vi "Multiple Connections - Server - TCP - 複製 (2).vi"() -> ()   [LabVIEW 2011]
doc: "Demonstrates how to establish multiple connections and place them in a queue to be serviced. As connections are made, it sends the current date and time via TCP to all Client VIs that connect to it.\n\nThis VI has two parts -- a loop that listens for each client to connect, and a loop that sends the date and time to each connection in the queue.\n\n<B>Note:</B> Use this VI with Multiple Connections - Client 1.vi and Multiple Connections - Client 2.vi."
panel:
  in  "Port 1":u16=6341
  in  "Port 2":u16=6342
  out "#2 Connections":i32
  out "#1 Connections":i32
  in  "stop":bool
  # "TCP Exchange V1.0"
  # "Internal Network"
  # "External Network"
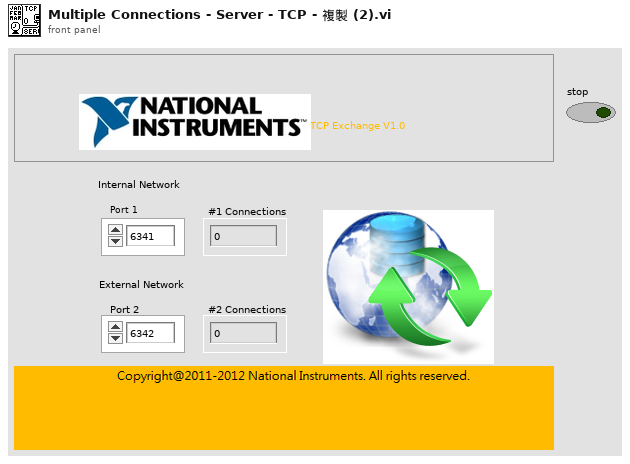
[diagram p1: front panel]
types:
  T1 = enum16{"Obtain", "Enqueue", "Dequeue", "Release"}
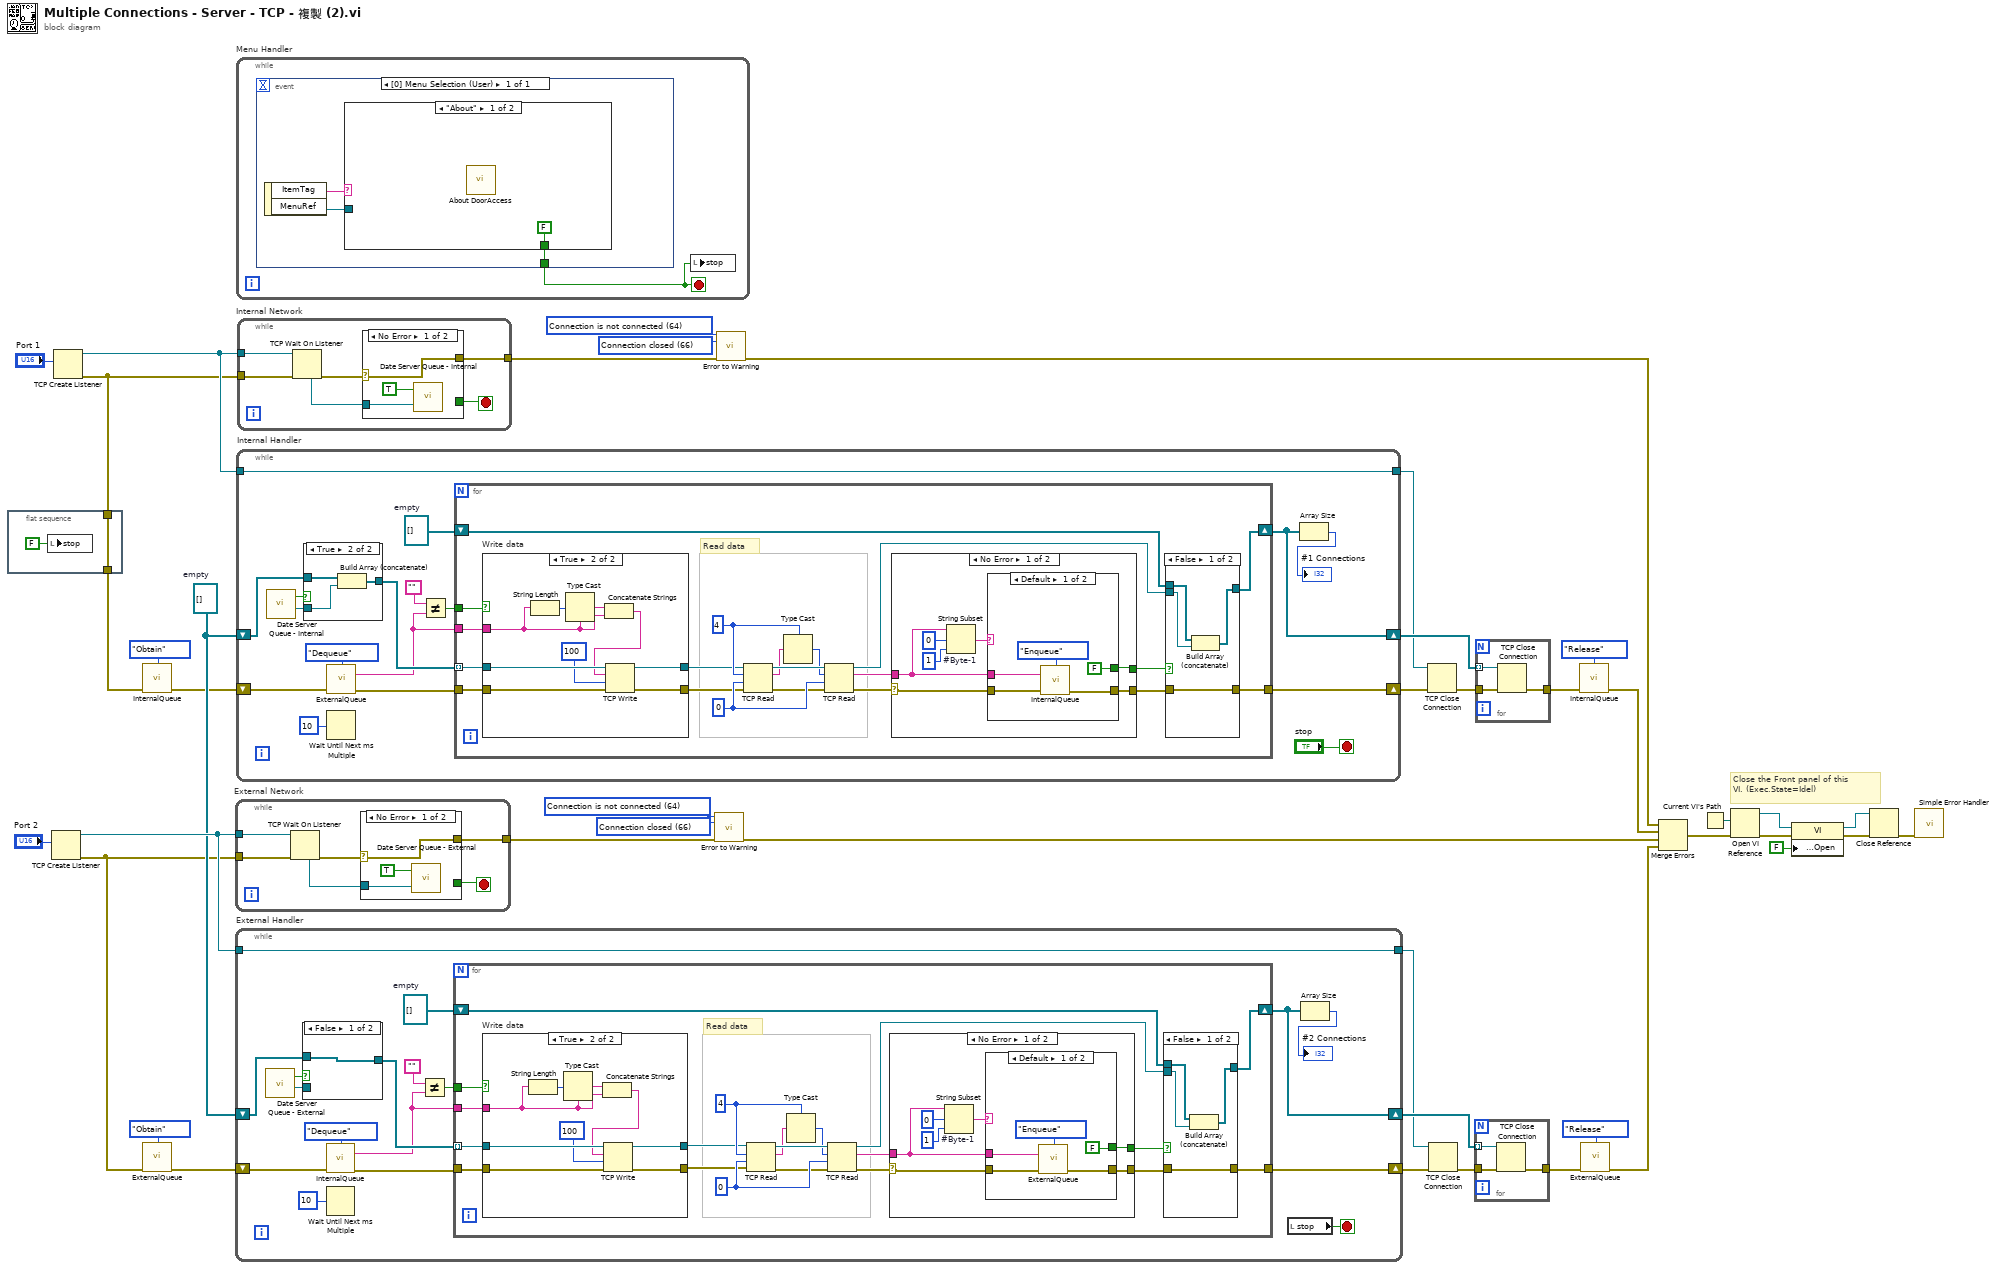
[diagram p0: block diagram]
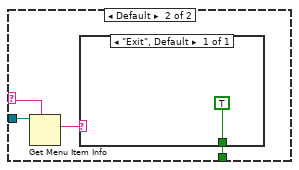
[diagram p2: hidden frame]
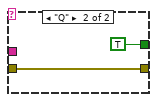
[diagram p3: hidden frame]
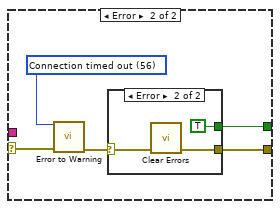
[diagram p4: hidden frame]
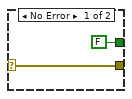
[diagram p5: hidden frame]
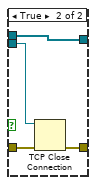
[diagram p7: hidden frame]
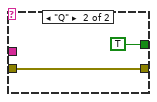
[diagram p9: hidden frame]
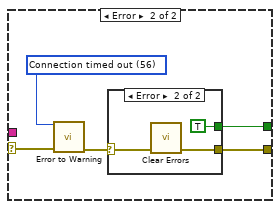
[diagram p10: hidden frame]
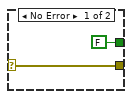
[diagram p11: hidden frame]
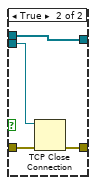
[diagram p13: hidden frame]
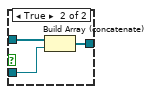
[diagram p14: hidden frame]
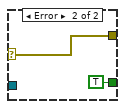
[diagram p15: hidden frame]
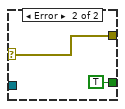
[diagram p16: hidden frame]
diagram:
  w31 = 66 items=["No Error", "Argument Error", "Memory Full", "Out of Zone", "End of File", "File Already Open", "Generic File IO Error", "File Not Found", "File Permission Error", "Disk Full", "Duplicate Path", "Too Many Files Open", "Not Enabled", "Resource File Not Found", "Cannot Add Resource", "Resource Not Found", "Image Not Found", "Image Memory Error", "Pen Does Not Exist", "Config Bad Type", "Config Token Not Found", "Config Parse Error", "Config Memory Error", "Bad External Code Format", "Bad External Code Offset", "External Code Not Present", "Null Window", "Destroy Window Mixup", "Null Menu", "Print Aborted", "Bad Print Record", "Print Driver Error", "Windows Error During Print", "Memory Error During Print", "Print Dialog Error", "Generic Print Error", "Invalid Device Refnum", "Device Not Found", "Device Parameter Error", "Device Unit Error", "Can't Open Device", "Device Call Aborted", "Generic Error", "Cancelled By User", "Object ID Too Low", "Object ID Too High", "Object Not In Heap", "Unknown Heap", "Bad DefProc ID", "DefProc Not In Table", "Message Out Of Range", "Null Method", "Unknown Message", "Manager Call Not Supported", "Bad address", "Connection In progress", "Connection timed out", "Connection is already in progress", "Network attribute not supported", "Network error", "Address in use", "System out of memory", "Connection aborted", "Connection refused", "Connection is not connected", "Connection is already connected", "Connection closed", "Initialize error (interapplication manager)", "Bad occurrence", "Wait on unbound occurrence handler", "Occurrence queue overflow", "Bad path", "Semaphore not signaled", "Unrecognized type (interapplication manager)"] ("2nd Error to Convert")
  w30 = 64 items=["No Error", "Argument Error", "Memory Full", "Out of Zone", "End of File", "File Already Open", "Generic File IO Error", "File Not Found", "File Permission Error", "Disk Full", "Duplicate Path", "Too Many Files Open", "Not Enabled", "Resource File Not Found", "Cannot Add Resource", "Resource Not Found", "Image Not Found", "Image Memory Error", "Pen Does Not Exist", "Config Bad Type", "Config Token Not Found", "Config Parse Error", "Config Memory Error", "Bad External Code Format", "Bad External Code Offset", "External Code Not Present", "Null Window", "Destroy Window Mixup", "Null Menu", "Print Aborted", "Bad Print Record", "Print Driver Error", "Windows Error During Print", "Memory Error During Print", "Print Dialog Error", "Generic Print Error", "Invalid Device Refnum", "Device Not Found", "Device Parameter Error", "Device Unit Error", "Can't Open Device", "Device Call Aborted", "Generic Error", "Cancelled By User", "Object ID Too Low", "Object ID Too High", "Object Not In Heap", "Unknown Heap", "Bad DefProc ID", "DefProc Not In Table", "Message Out Of Range", "Null Method", "Unknown Message", "Manager Call Not Supported", "Bad address", "Connection In progress", "Connection timed out", "Connection is already in progress", "Network attribute not supported", "Network error", "Address in use", "System out of memory", "Connection aborted", "Connection refused", "Connection is not connected", "Connection is already connected", "Connection closed", "Initialize error (interapplication manager)", "Bad occurrence", "Wait on unbound occurrence handler", "Occurrence queue overflow", "Bad path", "Semaphore not signaled", "Unrecognized type (interapplication manager)"] ("1st Error to Convert")
  w15 = refnum<k5>[] []  # empty
  w40 = 66 items=["No Error", "Argument Error", "Memory Full", "Out of Zone", "End of File", "File Already Open", "Generic File IO Error", "File Not Found", "File Permission Error", "Disk Full", "Duplicate Path", "Too Many Files Open", "Not Enabled", "Resource File Not Found", "Cannot Add Resource", "Resource Not Found", "Image Not Found", "Image Memory Error", "Pen Does Not Exist", "Config Bad Type", "Config Token Not Found", "Config Parse Error", "Config Memory Error", "Bad External Code Format", "Bad External Code Offset", "External Code Not Present", "Null Window", "Destroy Window Mixup", "Null Menu", "Print Aborted", "Bad Print Record", "Print Driver Error", "Windows Error During Print", "Memory Error During Print", "Print Dialog Error", "Generic Print Error", "Invalid Device Refnum", "Device Not Found", "Device Parameter Error", "Device Unit Error", "Can't Open Device", "Device Call Aborted", "Generic Error", "Cancelled By User", "Object ID Too Low", "Object ID Too High", "Object Not In Heap", "Unknown Heap", "Bad DefProc ID", "DefProc Not In Table", "Message Out Of Range", "Null Method", "Unknown Message", "Manager Call Not Supported", "Bad address", "Connection In progress", "Connection timed out", "Connection is already in progress", "Network attribute not supported", "Network error", "Address in use", "System out of memory", "Connection aborted", "Connection refused", "Connection is not connected", "Connection is already connected", "Connection closed", "Initialize error (interapplication manager)", "Bad occurrence", "Wait on unbound occurrence handler", "Occurrence queue overflow", "Bad path", "Semaphore not signaled", "Unrecognized type (interapplication manager)"] ("2nd Error to Convert")
  w41 = 64 items=["No Error", "Argument Error", "Memory Full", "Out of Zone", "End of File", "File Already Open", "Generic File IO Error", "File Not Found", "File Permission Error", "Disk Full", "Duplicate Path", "Too Many Files Open", "Not Enabled", "Resource File Not Found", "Cannot Add Resource", "Resource Not Found", "Image Not Found", "Image Memory Error", "Pen Does Not Exist", "Config Bad Type", "Config Token Not Found", "Config Parse Error", "Config Memory Error", "Bad External Code Format", "Bad External Code Offset", "External Code Not Present", "Null Window", "Destroy Window Mixup", "Null Menu", "Print Aborted", "Bad Print Record", "Print Driver Error", "Windows Error During Print", "Memory Error During Print", "Print Dialog Error", "Generic Print Error", "Invalid Device Refnum", "Device Not Found", "Device Parameter Error", "Device Unit Error", "Can't Open Device", "Device Call Aborted", "Generic Error", "Cancelled By User", "Object ID Too Low", "Object ID Too High", "Object Not In Heap", "Unknown Heap", "Bad DefProc ID", "DefProc Not In Table", "Message Out Of Range", "Null Method", "Unknown Message", "Manager Call Not Supported", "Bad address", "Connection In progress", "Connection timed out", "Connection is already in progress", "Network attribute not supported", "Network error", "Address in use", "System out of memory", "Connection aborted", "Connection refused", "Connection is not connected", "Connection is already connected", "Connection closed", "Initialize error (interapplication manager)", "Bad occurrence", "Wait on unbound occurrence handler", "Occurrence queue overflow", "Bad path", "Semaphore not signaled", "Unrecognized type (interapplication manager)"] ("1st Error to Convert")
  # "Close the Front panel of this\nVI. (Exec.State=Idel)"
  n1 = flat-sequence {
    tunnel: [w43] -> w5
    tunnel: w4 -> [w43]
    frame #0 {
      n2 = local write "stop"(FALSE ("stop")) -> ()
    }
  }
  n3 = TCP Create Listener(10:"Port 2") -> (0:w12:errorcluster, 3:w28:refnum<k5>)  [unwired: 1 in, 4 out]
  n4 = TCP Create Listener(10:"Port 1") -> (0:w4:errorcluster, 3:w16:refnum<k5>)  [unwired: 1 in, 4 out]
  n5 = call "InternalQueue.vi"("Mode"=T1."Obtain", "error in (no error)"=w5) -> ("error out"=w14:errorcluster)  [unwired: 12 in, 1 out]
  n6 = call "ExternalQueue.vi"("Mode"=T1."Obtain", "error in (no error)"=w12) -> ("error out"=w13:errorcluster)  [unwired: 12 in, 1 out]
  n7 = while "External Network" {
    tunnel: w28 -> [w49]
    tunnel: w12 -> [w50]
    tunnel: [w45] -> w29
    stop <- w46 stop-if-true
    n8 = TCP Wait On Listener(8:w50, 11:w49) -> (0:w47:errorcluster, 4:w48:refnum<k5>)  [unwired: 5 out]
    n9 = case shown="No Error" w47 {
      selector: w47 -> [w51 w54]
      tunnel: w48 -> [w52 _]
      tunnel: [_ TRUE] -> w46
      tunnel: [w51 w54] -> w45
      frame No Error {
        n10 = call "Date Server Queue - External.vi"("new value"=w52, "set queue? (F: de-queue)"=TRUE) -> ()  [unwired: 2 out]
      }
      frame Error {
      }
    }
  }
  n11 = while "External Handler" {
    shift-left: w15 -> [w70]
    shift-right: [w67] -> w27
    tunnel: w28 -> [w66]
    tunnel: [w66] -> w2
    shift-right: [w65] -> w34
    shift-left: w13 -> [w63]
    stop <- w61 stop-if-true
    w68 = refnum<k5>[] []  # empty
    n12 = call "Date Server Queue - External.vi"() -> ("value"=w72:refnum<k5>, "valid?"=w71:bool)  [unwired: 2 in]
    n13 = case shown="False" w71 {
      tunnel: w72 -> [_ w139]
      tunnel: w70 -> [w136 w138]
      tunnel: [w136 w137] -> w69
      frame False {
      }
      frame True {
        n14 = Build Array (concatenate)(w138, w139) -> (w137:refnum<k5>[])
      }
    }
    n15 = call "InternalQueue.vi"("Mode"=T1."Dequeue", "error in (no error)"=w63) -> ("Queue Out"=w58:string, "error out"=w62:errorcluster)  [unwired: 12 in]
    n16 = Wait Until Next ms Multiple(millisecond multiple=u32 10) -> ()  [unwired: 1 out]
    n17 = Not Equal?(x="", y=w58) -> (x != y?=w57:bool)
    n18 = for {
      tunnel: w69 -> [w89] mode=indexing
      shift-right: [w90] -> w67
      shift-left: w68 -> [w92]
      tunnel: [w91] -> w65
      tunnel: w62 -> [w88]
      tunnel: w58 -> [w85]
      tunnel: w57 -> [w84]
      w83 = 0 ("timeout ms (25000)")
      w81 = 4
      # "Read data"
      n19 = case "Write data" shown="True" w84 {
        tunnel: w89 -> [w118 w123]
        tunnel: w88 -> [w117 w125]
        tunnel: [w117 w121] -> w73
        tunnel: w85 -> [_ w124]
        tunnel: [w118 w119] -> w74
        frame False {
        }
        frame True {
          n20 = String Length(string=w124) -> (length=w127:i32)
          n21 = Type Cast(type=w124, x=w127) -> (*(type *) &x=w126:string)
          n22 = Concatenate Strings(w126, w124) -> (w120:string)
          n23 = TCP Write(connection ID=w123, data in=w120, error in (no error)=w125, 9:100 ("timeout ms (25000)")) -> (connection ID out=w119:refnum<k5>, error out=w121:errorcluster)  [unwired: 1 out]
        }
      }
      n24 = TCP Read(connection ID=w74, bytes to read=w81, error in (no error)=w73, 9:w83) -> (connection ID out=w82:refnum<k5>, data out=w80:string, error out=w79:errorcluster)  [unwired: 1 out]
      n25 = Type Cast(type=w81, x=w80) -> (*(type *) &x=w78:i32)
      n26 = TCP Read(connection ID=w82, bytes to read=w78, error in (no error)=w79, 9:w83) -> (connection ID out=w77:refnum<k5>, data out=w76:string, error out=w75:errorcluster)  [unwired: 1 out]
      n27 = case shown="No Error" w75 {
        selector: w75 -> [w95 w111]
        tunnel: [w94 w108] -> w86
        tunnel: [w93 w107] -> w87
        tunnel: w76 -> [w96 _]
        frame No Error {
          n28 = String Subset "#Byte-1"(string=w96, offset (0)=0, length (rest)=1 ("length (rest)")) -> (substring=w97:string)
          n29 = case shown="Default" w97 {
            tunnel: w96 -> [w100 _]
            tunnel: w95 -> [w102 w106]
            tunnel: [w101 w106] -> w94
            tunnel: [FALSE TRUE] -> w93
            frame Default {
              n30 = call "ExternalQueue.vi"("Mode"=T1."Enqueue", "Queue In"=w100, "error in (no error)"=w102) -> ("error out"=w101:errorcluster)  [unwired: 11 in, 1 out]
            }
            frame "Q" {
            }
          }
        }
        frame Error {
          w110 = 56 items=["No Error", "Argument Error", "Memory Full", "Out of Zone", "End of File", "File Already Open", "Generic File IO Error", "File Not Found", "File Permission Error", "Disk Full", "Duplicate Path", "Too Many Files Open", "Not Enabled", "Resource File Not Found", "Cannot Add Resource", "Resource Not Found", "Image Not Found", "Image Memory Error", "Pen Does Not Exist", "Config Bad Type", "Config Token Not Found", "Config Parse Error", "Config Memory Error", "Bad External Code Format", "Bad External Code Offset", "External Code Not Present", "Null Window", "Destroy Window Mixup", "Null Menu", "Print Aborted", "Bad Print Record", "Print Driver Error", "Windows Error During Print", "Memory Error During Print", "Print Dialog Error", "Generic Print Error", "Invalid Device Refnum", "Device Not Found", "Device Parameter Error", "Device Unit Error", "Can't Open Device", "Device Call Aborted", "Generic Error", "Cancelled By User", "Object ID Too Low", "Object ID Too High", "Object Not In Heap", "Unknown Heap", "Bad DefProc ID", "DefProc Not In Table", "Message Out Of Range", "Null Method", "Unknown Message", "Manager Call Not Supported", "Bad address", "Connection In progress", "Connection timed out", "Connection is already in progress", "Network attribute not supported", "Network error", "Address in use", "System out of memory", "Connection aborted", "Connection refused", "Connection is not connected", "Connection is already connected", "Connection closed", "Initialize error (interapplication manager)", "Bad occurrence", "Wait on unbound occurrence handler", "Occurrence queue overflow", "Bad path", "Semaphore not signaled", "Unrecognized type (interapplication manager)"] ("1st Error to Convert")
          n31 = call <vilib>:"Error to Warning.vi"("1st Error to Convert"=w110, "error in"=w111) -> ("warning out"=w109:errorcluster)  [unwired: 13 in]
          n32 = case shown="Error" w109 {
            selector: w109 -> [w113 w116]
            tunnel: [w113 w115] -> w108
            tunnel: [FALSE TRUE] -> w107
            frame No Error {
            }
            frame Error {
              n33 = call <vilib>:"Clear Errors.vi"("error in (no error)"=w116) -> ("error out"=w115:errorcluster)  [unwired: 6 in]
            }
          }
        }
      }
      n34 = case shown="False" w87 {
        tunnel: w92 -> [w131 w135]
        tunnel: w77 -> [w130 w134]
        tunnel: [w129 w135] -> w90
        tunnel: w86 -> [w128 w133]
        tunnel: [w128 w132] -> w91
        frame False {
          n35 = Build Array (concatenate)(w131, w130) -> (w129:refnum<k5>[])
        }
        frame True {
          n36 = TCP Close Connection(connection ID=w134, error in (no error)=w133) -> (error out=w132:errorcluster)  [unwired: 2 out]
        }
      }
    }
    n37 = local read "stop"() -> (w61:bool)
    n38 = Array Size(array=w67) -> (size(s)=→"#2 Connections":i32)
  }
  n39 = while "Menu Handler" {
    stop <- w140 stop-if-true
    n40 = event shown="[0] Menu Selection (User)" {
      selector: _ -> [_]
      dyn-events: _ -> [_]
      timeout: _ -> [_]
      tunnel: [w141] -> w140
      event Menu Selection (User) {
        n41 = event-data() -> ("ItemTag"=w142:string, "MenuRef"=w143:refnum<k9>)  [unwired: 1 in]
        n42 = case shown="\"About\"" w142 {
          selector: w142 -> [_ w147]
          tunnel: w143 -> [_ w148]
          tunnel: [FALSE w145] -> w141
          frame "About" {
            n43 = call "About DoorAccess.vi"() -> ()  [unwired: 1 out]
          }
          frame Default {
            n44 = Get Menu Item Info(7:w147, 11:w148) -> (2:w146:string)  [unwired: 1 in, 6 out]
            n45 = case shown="\"Exit\", Default" w146 {
              tunnel: [TRUE] -> w145
              frame "Exit", Default {
              }
            }
          }
        }
      }
    }
    n46 = local write "stop"(w140) -> ()
  }
  n47 = while "Internal Handler" {
    shift-left: w15 -> [w164]
    shift-right: [w161] -> w17
    tunnel: w16 -> [w160]
    tunnel: [w160] -> w1
    shift-right: [w159] -> w18
    shift-left: w14 -> [w157]
    stop <- "stop" stop-if-true
    w162 = refnum<k5>[] []  # empty
    n48 = call "Date Server Queue - Internal.vi"() -> ("value"=w166:refnum<k5>, "valid?"=w165:bool)  [unwired: 2 in]
    n49 = case shown="True" w165 {
      tunnel: w166 -> [_ w233]
      tunnel: w164 -> [w230 w232]
      tunnel: [w230 w231] -> w163
      frame False {
      }
      frame True {
        n50 = Build Array (concatenate)(w232, w233) -> (w231:refnum<k5>[])
      }
    }
    n51 = call "ExternalQueue.vi"("Mode"=T1."Dequeue", "error in (no error)"=w157) -> ("Queue Out"=w153:string, "error out"=w156:errorcluster)  [unwired: 12 in]
    n52 = Wait Until Next ms Multiple(millisecond multiple=u32 10) -> ()  [unwired: 1 out]
    n53 = Not Equal?(x="", y=w153) -> (x != y?=w152:bool)
    n54 = for {
      tunnel: w163 -> [w183] mode=indexing
      shift-right: [w184] -> w161
      shift-left: w162 -> [w186]
      tunnel: [w185] -> w159
      tunnel: w156 -> [w182]
      tunnel: w153 -> [w179]
      tunnel: w152 -> [w178]
      w177 = 0 ("timeout ms (25000)")
      w175 = 4
      # "Read data"
      n55 = case "Write data" shown="True" w178 {
        tunnel: w183 -> [w212 w217]
        tunnel: w182 -> [w211 w219]
        tunnel: [w211 w215] -> w171
        tunnel: w179 -> [_ w218]
        tunnel: [w212 w213] -> w170
        frame False {
        }
        frame True {
          n56 = String Length(string=w218) -> (length=w221:i32)
          n57 = Type Cast(type=w218, x=w221) -> (*(type *) &x=w220:string)
          n58 = Concatenate Strings(w220, w218) -> (w214:string)
          n59 = TCP Write(connection ID=w217, data in=w214, error in (no error)=w219, 9:100 ("timeout ms (25000)")) -> (connection ID out=w213:refnum<k5>, error out=w215:errorcluster)  [unwired: 1 out]
        }
      }
      n60 = TCP Read(connection ID=w170, bytes to read=w175, error in (no error)=w171, 9:w177) -> (connection ID out=w176:refnum<k5>, data out=w174:string, error out=w173:errorcluster)  [unwired: 1 out]
      n61 = Type Cast(type=w175, x=w174) -> (*(type *) &x=w172:i32)
      n62 = TCP Read(connection ID=w176, bytes to read=w172, error in (no error)=w173, 9:w177) -> (connection ID out=w169:refnum<k5>, data out=w167:string, error out=w168:errorcluster)  [unwired: 1 out]
      n63 = case shown="No Error" w168 {
        selector: w168 -> [w189 w205]
        tunnel: [w188 w202] -> w180
        tunnel: [w187 w201] -> w181
        tunnel: w167 -> [w190 _]
        frame No Error {
          n64 = String Subset "#Byte-1"(string=w190, offset (0)=0, length (rest)=1 ("length (rest)")) -> (substring=w191:string)
          n65 = case shown="Default" w191 {
            tunnel: w190 -> [w194 _]
            tunnel: w189 -> [w196 w200]
            tunnel: [w195 w200] -> w188
            tunnel: [FALSE TRUE] -> w187
            frame Default {
              n66 = call "InternalQueue.vi"("Mode"=T1."Enqueue", "Queue In"=w194, "error in (no error)"=w196) -> ("error out"=w195:errorcluster)  [unwired: 11 in, 1 out]
            }
            frame "Q" {
            }
          }
        }
        frame Error {
          w204 = 56 items=["No Error", "Argument Error", "Memory Full", "Out of Zone", "End of File", "File Already Open", "Generic File IO Error", "File Not Found", "File Permission Error", "Disk Full", "Duplicate Path", "Too Many Files Open", "Not Enabled", "Resource File Not Found", "Cannot Add Resource", "Resource Not Found", "Image Not Found", "Image Memory Error", "Pen Does Not Exist", "Config Bad Type", "Config Token Not Found", "Config Parse Error", "Config Memory Error", "Bad External Code Format", "Bad External Code Offset", "External Code Not Present", "Null Window", "Destroy Window Mixup", "Null Menu", "Print Aborted", "Bad Print Record", "Print Driver Error", "Windows Error During Print", "Memory Error During Print", "Print Dialog Error", "Generic Print Error", "Invalid Device Refnum", "Device Not Found", "Device Parameter Error", "Device Unit Error", "Can't Open Device", "Device Call Aborted", "Generic Error", "Cancelled By User", "Object ID Too Low", "Object ID Too High", "Object Not In Heap", "Unknown Heap", "Bad DefProc ID", "DefProc Not In Table", "Message Out Of Range", "Null Method", "Unknown Message", "Manager Call Not Supported", "Bad address", "Connection In progress", "Connection timed out", "Connection is already in progress", "Network attribute not supported", "Network error", "Address in use", "System out of memory", "Connection aborted", "Connection refused", "Connection is not connected", "Connection is already connected", "Connection closed", "Initialize error (interapplication manager)", "Bad occurrence", "Wait on unbound occurrence handler", "Occurrence queue overflow", "Bad path", "Semaphore not signaled", "Unrecognized type (interapplication manager)"] ("1st Error to Convert")
          n67 = call <vilib>:"Error to Warning.vi"("1st Error to Convert"=w204, "error in"=w205) -> ("warning out"=w203:errorcluster)  [unwired: 13 in]
          n68 = case shown="Error" w203 {
            selector: w203 -> [w207 w210]
            tunnel: [w207 w209] -> w202
            tunnel: [FALSE TRUE] -> w201
            frame No Error {
            }
            frame Error {
              n69 = call <vilib>:"Clear Errors.vi"("error in (no error)"=w210) -> ("error out"=w209:errorcluster)  [unwired: 6 in]
            }
          }
        }
      }
      n70 = case shown="False" w181 {
        tunnel: w186 -> [w225 w229]
        tunnel: w169 -> [w224 w228]
        tunnel: [w223 w229] -> w184
        tunnel: w180 -> [w222 w227]
        tunnel: [w222 w226] -> w185
        frame False {
          n71 = Build Array (concatenate)(w225, w224) -> (w223:refnum<k5>[])
        }
        frame True {
          n72 = TCP Close Connection(connection ID=w228, error in (no error)=w227) -> (error out=w226:errorcluster)  [unwired: 2 out]
        }
      }
    }
    n73 = Array Size(array=w161) -> (size(s)=→"#1 Connections":i32)
  }
  n74 = while "Internal Network" {
    tunnel: w16 -> [w238]
    tunnel: w4 -> [w239]
    tunnel: [w234] -> w42
    stop <- w235 stop-if-true
    n75 = TCP Wait On Listener(8:w239, 11:w238) -> (0:w236:errorcluster, 4:w237:refnum<k5>)  [unwired: 5 out]
    n76 = case shown="No Error" w236 {
      selector: w236 -> [w240 w243]
      tunnel: w237 -> [w241 _]
      tunnel: [_ TRUE] -> w235
      tunnel: [w240 w243] -> w234
      frame No Error {
        n77 = call "Date Server Queue - Internal.vi"("new value"=w241, "set queue? (F: de-queue)"=TRUE) -> ()  [unwired: 2 out]
      }
      frame Error {
      }
    }
  }
  n78 = call <vilib>:"Error to Warning.vi"("1st Error to Convert"=w30, "2nd Error to Convert"=w31, "error in"=w29) -> ("warning out"=w26:errorcluster)  [unwired: 2 in, 10 out]
  n79 = call <vilib>:"Error to Warning.vi"("1st Error to Convert"=w41, "2nd Error to Convert"=w40, "error in"=w42) -> ("warning out"=w37:errorcluster)  [unwired: 2 in, 10 out]
  n80 = TCP Close Connection(connection ID=w1, error in (no error)=w18) -> (error out=w38:errorcluster)  [unwired: 2 out]
  n81 = TCP Close Connection(connection ID=w2, error in (no error)=w34) -> (error out=w33:errorcluster)  [unwired: 2 out]
  n82 = for {
    tunnel: w27 -> [w247] mode=indexing
    tunnel: [w246] -> w8
    tunnel: w33 -> [w245]
    n83 = TCP Close Connection(connection ID=w247, error in (no error)=w245) -> (error out=w246:errorcluster)  [unwired: 2 out]
  }
  n84 = for {
    tunnel: w17 -> [w250] mode=indexing
    tunnel: [w249] -> w10
    tunnel: w38 -> [w248]
    n85 = TCP Close Connection(connection ID=w250, error in (no error)=w248) -> (error out=w249:errorcluster)  [unwired: 2 out]
  }
  n86 = call "InternalQueue.vi"("Mode"=T1."Release", "error in (no error)"=w10) -> ("error out"=w9:errorcluster)  [unwired: 12 in, 1 out]
  n87 = call "ExternalQueue.vi"("Mode"=T1."Release", "error in (no error)"=w8) -> ("error out"=w7:errorcluster)  [unwired: 12 in, 1 out]
  n88 = Merge Errors(w37, w9, w26, w7) -> (w3:errorcluster)
  n89 = Current VI's Path() -> (path=w25:path)
  n90 = Open VI Reference(vi path=w25, error in (no error)=w3) -> (vi reference=w20:refnum<vi>, error out=w24:errorcluster)  [unwired: 4 in]
  n91 = property class="VI"(reference=w20, error in=w24, "Front Panel Window:Open"=FALSE) -> (reference out=w23:refnum<vi>, error out=w21:errorcluster)
  n92 = Close Reference(reference=w23, error in (no error)=w21) -> (error out=w19:errorcluster)
  n93 = call <vilib>:"Simple Error Handler.vi"("error in (no error)"=w19) -> ()  [unwired: 1 in, 8 out]
